vi "Global mqttExample.vi"() -> ()   [LabVIEW 2017]
panel:
  in  "send client time":bool
  out "MQTT Connection":bool
  out "quit":bool
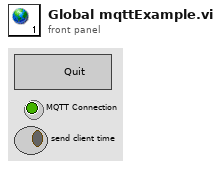
[diagram p1: front panel]
diagram:
